vi "S2C_FORNAX_Proc_ReleaseQs.vi"(8 "Error In":errorcluster, 11 "Q-Ref":refnum<queue>) -> (0 "Error Out":errorcluster)   [LabVIEW 2015]
uses:
  S2C_FORNAX_Proc_Globals.vi
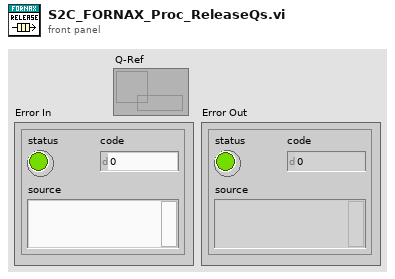
[diagram p1: front panel]
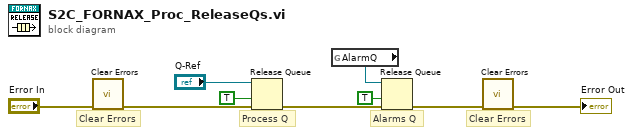
[diagram p0: block diagram]
diagram:
  # "Clear Errors"
  # "Clear Errors"
  # "Alarms Q"
  # "Process Q"
  n1 = call <vilib>:"Clear Errors.vi"("error in (no error)"="Error In") -> ("error out"=w1:errorcluster)  [unwired: 5 in, 1 out]
  n2 = Release Queue(queue="Q-Ref", force destroy? (F)=TRUE, error in (no error)=w1) -> (error out=w5:errorcluster)  [unwired: 2 out]
  n3 = global read "S2C_FORNAX_Proc_Globals.vi" "AlarmQ"() -> (w4:refnum<queue>)
  n4 = Release Queue(queue=w4, force destroy? (F)=TRUE, error in (no error)=w5) -> (error out=w2:errorcluster)  [unwired: 2 out]
  n5 = call <vilib>:"Clear Errors.vi"("error in (no error)"=w2) -> ("error out"=→"Error Out":errorcluster)  [unwired: 5 in, 1 out]
